vi "reports.vi"(7 "httpRequestID":u32, 9 "Debug":bool) -> ()   [LabVIEW 2014]
uses:
  FRCts20_EspEngine.lvlib
  <vilib>/wsapi/NI_WebServices.lvlib
  <vilib>/wsapi/subVIs/Set Boolean ESP Variable.vi
  TypeDefs/FRCts20_EspEngine_SwUsage_Pie.ctl
  TypeDefs/FRCts20_EspEngine_RequestPerHour_Line.ctl
  TypeDefs/FRCts20_EspEngine_AdvancedComponents_Bar.ctl
panel:
  in  "Advanced Components":T1={"CAN"=100, "Vision"=202, "Kinect"=151}
  in  "RequestsPerHour":T2={"StartDate"={"Year"=2012, "Month"=6, "Day"=15}, "Events"=[{"Location"="NYC", "Requests"=[5, 7, 6, 4]}, {"Location"="SF", "Requests"=[1, 3, 6, 5]}]}
  in  "SW Usage Pies":T3=[{"Live Event Location"="GLOBAL", "LabVIEW"=55.1, "C++"=15.1, "Java"=24.9, "Other"=4.9, "TotalTeams"=1000, "TeamsReporting"=900}, {"Live Event Location"="New York City", "LabVIEW"=54.0, "C++"=15.0, "Java"=16.0, "Other"=15.0, "TotalTeams"=65, "TeamsReporting"=63}, {"Live Event Location"="San Fransisco", "LabVIEW"=85.0, "C++"=5.0, "Java"=5.0, "Other"=5.0, "TotalTeams"=50, "TeamsReporting"=35}]
  out "error out":errorcluster
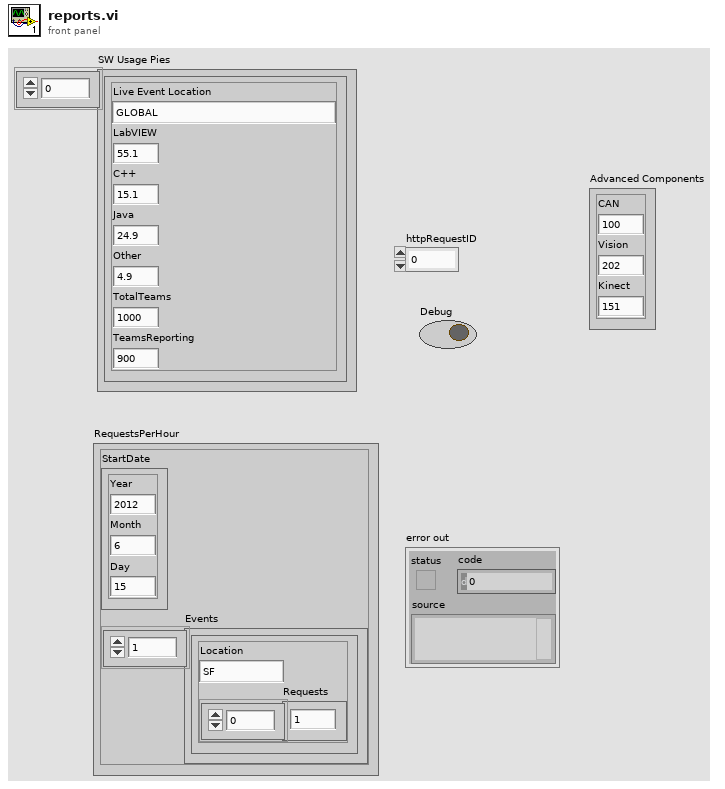
[diagram p1: front panel]
types:
  T1 = typedef "FRCts20_EspEngine.lvlib/FRCts20_EspEngine_AdvancedComponents_Bar.ctl" = cluster{"CAN":i32, "Vision":i32, "Kinect":i32}
  T2 = typedef "FRCts20_EspEngine.lvlib/FRCts20_EspEngine_RequestPerHour_Line.ctl" = cluster{"StartDate":cluster{"Year":i32, "Month":i32, "Day":i32}, "Events":cluster{"Location":string, "Requests":i32[]}[]}
  T3 = typedef "FRCts20_EspEngine.lvlib/FRCts20_EspEngine_SwUsage_Pie.ctl" = cluster{"Live Event Location":string, "LabVIEW":dbl, "C++":dbl, "Java":dbl, "Other":dbl, "TotalTeams":i32, "TeamsReporting":i32}[]
  T4 = typedef "FRCts20_EspEngine.lvlib/FRCts20_EspEngine_SearchBrowser.ctl" = cluster{"Event":cluster{"Event Index":u32, "Event Name":string, "Start Time":timestamp, "End Time":timestamp, "OpenIssues":u8, "IsLive":bool}[], "select-choice-software":string, "select-choice-location":string}
  T5 = cluster{"SW Usage Pies":T3, "RequestsPerHour":T2, "Advanced Components":T1}
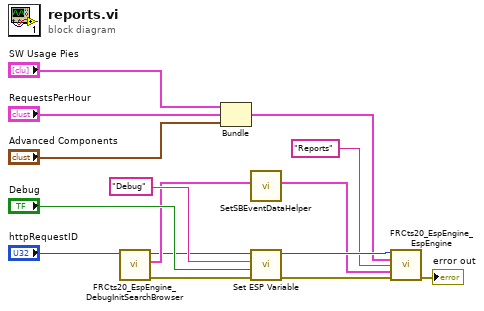
[diagram p0: block diagram]
diagram:
  n1 = call "FRCts20_EspEngine_DebugInitSearchBrowser.vi"("httpRequestID"="httpRequestID") -> ("error out"=w3:errorcluster, "SearchBrowser"=w5:T4, "httpRequestID out"=w1:u32)  [unwired: 8 in]
  n2 = Bundle("SW Usage Pies"="SW Usage Pies", "RequestsPerHour"="RequestsPerHour", "Advanced Components"="Advanced Components") -> (w7:T5)  [unwired: 1 in]
  n3 = call "SetSBEventDataHelper.vi"("SearchBrowser"=w5) -> ("SearchBrowser"=w4:T4)  [unwired: 10 in]
  n4 = call-poly <vilib>:"Set ESP Variable.vi"("error in (no error)"=w3, "value"="Debug", "key"="Debug", "httpRequestID"=w1) -> ("error out"=w10:errorcluster, "httpRequestID out"=w13:u32)  [unwired: 6 in]
  n5 = call "FRCts20_EspEngine_EspEngine.vi"("httpRequestID"=w13, "Cluster"=w7, "Page"="Reports", "SearchBrowser"=w4, "error in (no error)"=w10) -> ("error out"=→"error out":errorcluster)  [unwired: 9 in, 1 out]
